vi "Get 3D Map Data (no color).vi"(2 "Focal Length in Pixels":dbl, 3 "Remove Zeros?":bool, 4 "Depth Image Pixels (U16) In":u16[][](array[numeric])) -> (0 "3D Information Cluster (X,Y,Z)":cluster{dbl[], dbl[], dbl[]}, 1 "3D Information (X,Y,Z)":cluster{"x":dbl, "y":dbl, "z":dbl}[](array[cluster]))   [LabVIEW 2010, in "Kinect_API.lvlib"]
uses:
  Kinect_API.lvlib
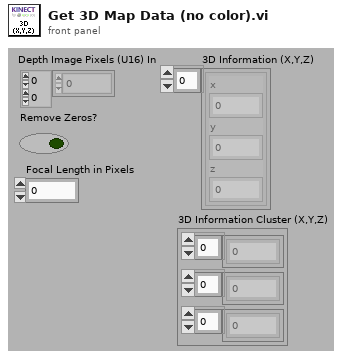
[diagram p1: front panel]
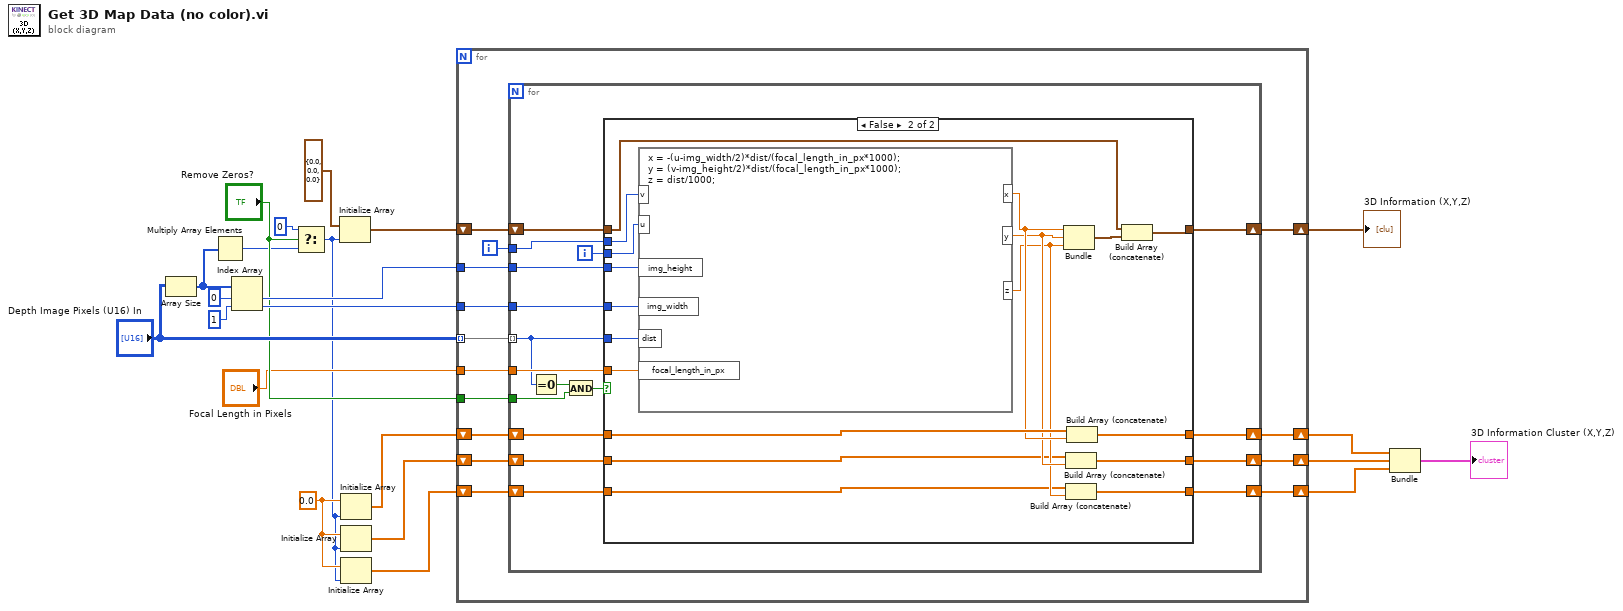
[diagram p0: block diagram]
diagram:
  w9 = 0.0 ("x")
  n1 = Array Size(array="Depth Image Pixels (U16) In") -> (size(s)=w12:i32[])
  n2 = Multiply Array Elements(1:w12) -> (0:w11:i32)
  n3 = Index Array(array=w12, index #1=0 ("index"), index #2=1 ("index")) -> (element #1=w19:i32, element #2=w20:i32)
  n4 = Select(t=0 ("dimension size"), s="Remove Zeros?", f=w11) -> (s? t:f=w8:i32)
  n5 = Initialize Array(cluster{"x":dbl, "y":dbl, "z":dbl} {"x"=0.0, "y"=0.0, "z"=0.0} ("output cluster"), w8) -> (w16:cluster{"x":dbl, "y":dbl, "z":dbl}[])
  n6 = Initialize Array(w9, w8) -> (w7:dbl[])
  n7 = Initialize Array(w9, w8) -> (w6:dbl[])
  n8 = Initialize Array(w9, w8) -> (w5:dbl[])
  n9 = for {
    tunnel: "Depth Image Pixels (U16) In" -> [w36] mode=indexing
    tunnel: w19 -> [w34]
    tunnel: w20 -> [w33]
    tunnel: "Focal Length in Pixels" -> [w32]
    shift-right: [w30] -> w15
    shift-left: w16 -> [w31]
    tunnel: "Remove Zeros?" -> [w29]
    shift-right: [w24] -> w3
    shift-left: w6 -> [w27]
    shift-right: [w25] -> w4
    shift-left: w7 -> [w28]
    shift-right: [w23] -> w2
    shift-left: w5 -> [w26]
    i -> [w35]
    n10 = for {
      tunnel: w36 -> [w46] mode=indexing
      tunnel: w35 -> [w53]
      tunnel: w34 -> [w51]
      tunnel: w33 -> [w50]
      tunnel: w32 -> [w47]
      shift-right: [w48] -> w30
      shift-left: w31 -> [w49]
      tunnel: w29 -> [w44]
      shift-right: [w38] -> w24
      shift-left: w27 -> [w41]
      shift-right: [w39] -> w25
      shift-left: w28 -> [w42]
      shift-right: [w37] -> w23
      shift-left: w26 -> [w40]
      i -> [w52]
      n11 = Equal To 0?(x=w46) -> (x = 0?=w45:bool)
      n12 = And(x=w45, y=w44) -> (x .and. y?=w43:bool)
      n13 = case shown="False" w43 {
        tunnel: w53 -> [_ w75]
        tunnel: w52 -> [_ w74]
        tunnel: w51 -> [_ w73]
        tunnel: w50 -> [_ w72]
        tunnel: w46 -> [_ w71]
        tunnel: w47 -> [_ w70]
        tunnel: w49 -> [w57 w68]
        tunnel: [w57 w67] -> w48
        tunnel: w42 -> [w56 w66]
        tunnel: w41 -> [w55 w62]
        tunnel: w40 -> [w54 w61]
        tunnel: [w56 w60] -> w39
        tunnel: [w55 w59] -> w38
        tunnel: [w54 w58] -> w37
        frame True {
        }
        frame False {
          n14 = formula code="x = -(u-img_width/2)*dist/(focal_length_in_px*1000);\ny = (v-img_height/2)*dist/(focal_length_in_px*1000);\nz = dist/1000;"("v"=w75, "u"=w74, "img_height"=w73, "img_width"=w72, "dist"=w71, "focal_length_in_px"=w70) -> ("x"=w65:dbl, "y"=w64:dbl, "z"=w63:dbl)
          n15 = Bundle("x"=w65, "y"=w64, "z"=w63) -> (w69:cluster{"x":dbl, "y":dbl, "z":dbl})  [unwired: 1 in]
          n16 = Build Array (concatenate)(w62, w64) -> (w59:dbl[])
          n17 = Build Array (concatenate)(w61, w63) -> (w58:dbl[])
          n18 = Build Array (concatenate)(w66, w65) -> (w60:dbl[])
          n19 = Build Array (concatenate)(w68, w69) -> (w67:cluster{"x":dbl, "y":dbl, "z":dbl}[])
        }
      }
    }
  }
  "3D Information (X,Y,Z)" <- w15
  n20 = Bundle(w4, w3, w2) -> (→"3D Information Cluster (X,Y,Z)":cluster{dbl[], dbl[], dbl[]})  [unwired: 1 in]
